vi "Write Key Value String.vi"(7 "Section Name":string, 8 "error in (no error)":errorcluster, 9 "Value":string, 10 "Key Name":string, 11 "ODBC-Interface in":refnum<class "ODBC-Interface.lvclass">) -> (0 "error out":errorcluster, 2 "found":bool, 3 "ODBC-Interface out":refnum<class "ODBC-Interface.lvclass">)   [LabVIEW 2014, in "DB-Configuration.lvlib" / "ODBC-Interface.lvclass"]
doc: "Write string key value."
uses:
  ODBC-Interface.lvclass
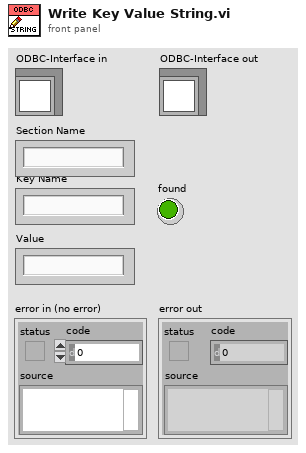
[diagram p1: front panel]
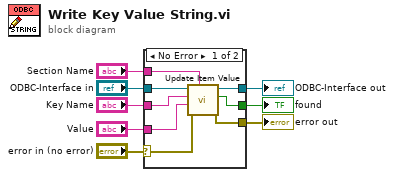
[diagram p0: block diagram]
diagram:
  n1 = case shown="No Error" "error in (no error)" {
    selector: "error in (no error)" -> [w10 w17]
    tunnel: "Section Name" -> [w16 _]
    tunnel: "ODBC-Interface in" -> [w15 w18]
    tunnel: [w14 w18] -> w3
    tunnel: "Key Name" -> [w13 _]
    tunnel: "Value" -> [w9 _]
    tunnel: [w12 w17] -> w1
    tunnel: [w11 _] -> w2
    frame No Error {
      n2 = call-dynamic "Update Item Value.vi"("Section Name"=w16, "error in (no error)"=w10, "Value"=w9, "Key Name"=w13, "ODBC-Interface in"=w15) -> ("error out"=w12:errorcluster, "found"=w11:bool, "ODBC-Interface out"=w14:refnum<class "ODBC-Interface.lvclass">)  [unwired: 4 in]
    }
    frame Error {
    }
  }
  "error out" <- w1
  "ODBC-Interface out" <- w3
  "found" <- w2
